vi "Beam Extraction.vi"() -> ()   [LabVIEW 2018]
uses:
  InstrumentStatusLib/com.insstat.lvlib
panel:
  out "?":bool
  out "?":bool
  out "?":bool
  out "?":bool
  out "?":string
  out "?":string
  out "?":string
  out "?":string
  out "?":bool
  out "?":bool
  out "?":bool
  out "?":bool
  out "?":string
  out "?":string
  out "?":string
  out "?":string
  out "Gate C":string
  out "Gate A":string
  out "REF":string
  out "Trig":string
  out "Gate B":string
  out "OUT":string
  out "Gate":string
  out "EN":string
  out "CS":string
  out "Pulse":string
  out "?":string
  out "?":string
  out "?":string
  out "?":string
  out "?":string
  out "?":string
  out "?":string
  out "?":string
  out "?":string
  out "?":string
  out "String":string
  out "?":string
  out "?":string
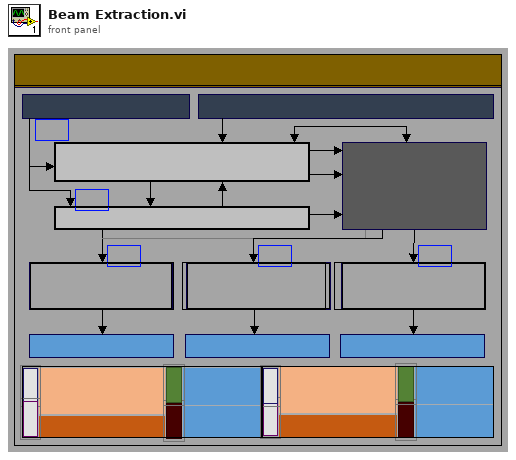
[diagram p1: front panel]
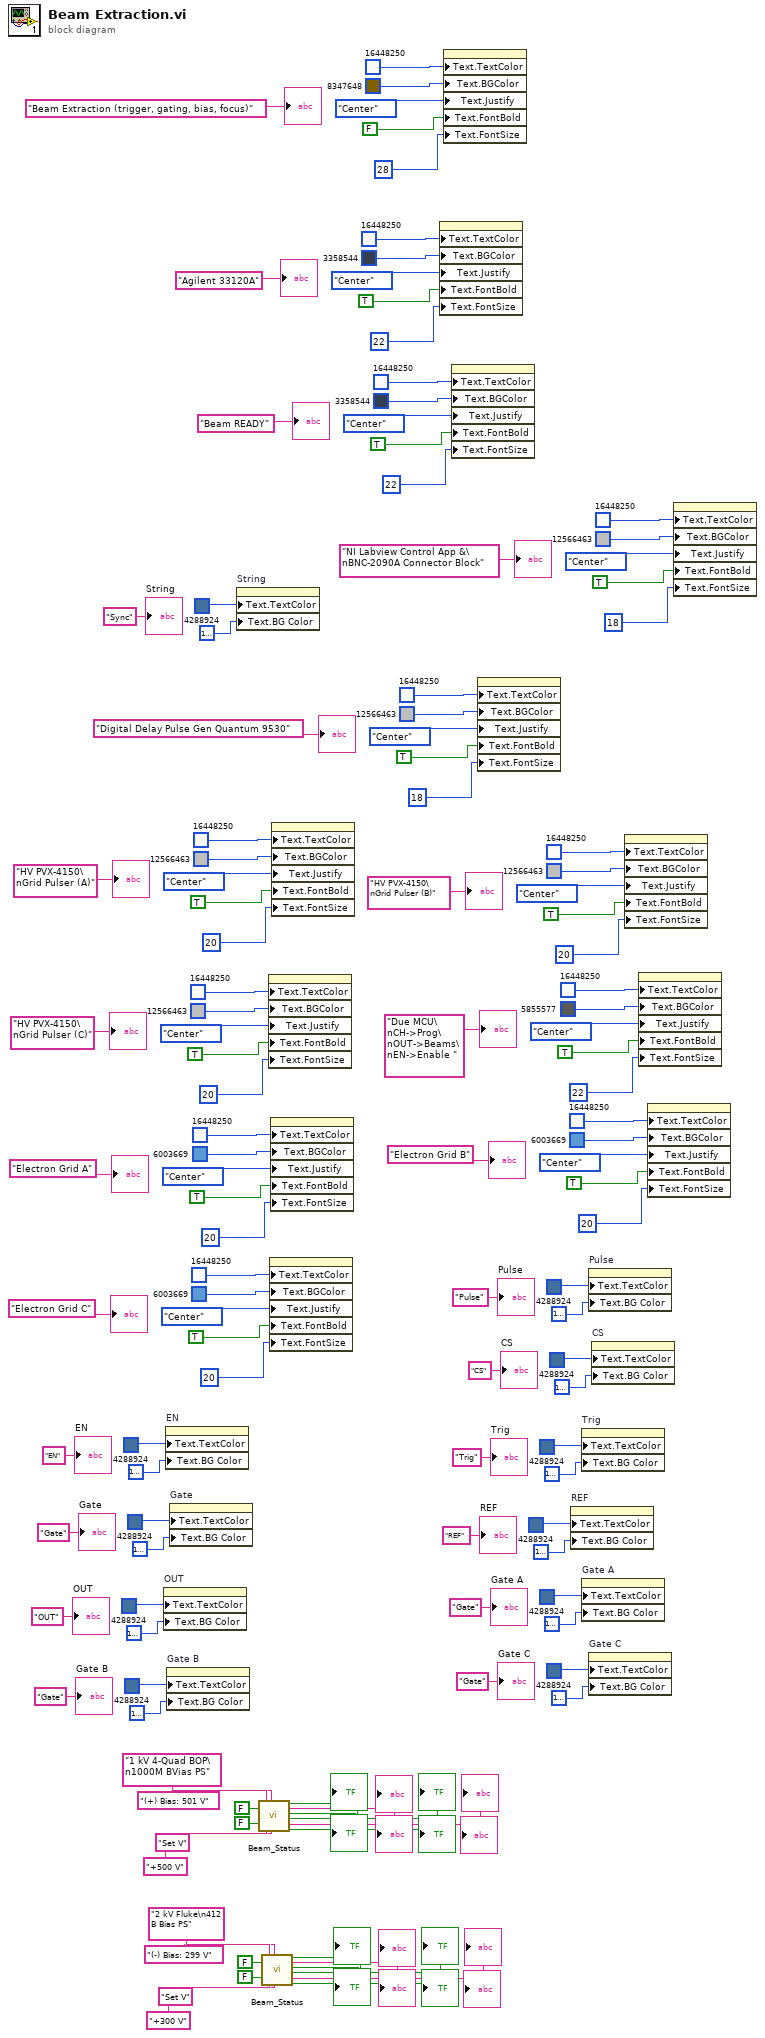
[diagram p0: block diagram]
diagram:
  n1 = property on="OUT" class="Str"("Text.TextColor"=u32 4288924, "Text.BG Color"=u32 16777216) -> ()  [unwired: 2 in, 2 out]
  n2 = property on="EN" class="Str"("Text.TextColor"=u32 4288924, "Text.BG Color"=u32 16777216) -> ()  [unwired: 2 in, 2 out]
  n3 = property on="Gate B" class="Str"("Text.TextColor"=u32 4288924, "Text.BG Color"=u32 16777216) -> ()  [unwired: 2 in, 2 out]
  n4 = property on="Gate" class="Str"("Text.TextColor"=u32 4288924, "Text.BG Color"=u32 16777216) -> ()  [unwired: 2 in, 2 out]
  n5 = property on="String" class="Str"("Text.TextColor"=u32 4288924, "Text.BG Color"=u32 16777216) -> ()  [unwired: 2 in, 2 out]
  n6 = call "Beam_Status.vi"("Power"=FALSE, "Activate"=FALSE, "String"="1 kV 4-Quad BOP\n1000M BVias PS", "String 3"="Set V", "String 2"="(+) Bias: 501 V", "String 4"="+500 V") -> (10:→"?":string, 11:→"?":string, 12:→"?":string, 13:→"?":string, 14:→"?":bool, 16:→"?":bool, 17:→"?":bool, 19:→"?":bool)  [unwired: 6 in]
  n7 = call "Beam_Status.vi"("Power"=FALSE, "Activate"=FALSE, "String"="2 kV Fluke\n412 B Bias PS", "String 3"="Set V", "String 2"="(-) Bias: 299 V", "String 4"="+300 V") -> (10:→"?":string, 11:→"?":string, 12:→"?":string, 13:→"?":string, 14:→"?":bool, 16:→"?":bool, 17:→"?":bool, 19:→"?":bool)  [unwired: 6 in]
  n8 = property class="Str"("Text.TextColor"=u32 16448250, "Text.BGColor"=u32 12566463, "Text.Justify"=enum16{"Left", "Center", "Right"}."Center" ("Text.Justification"), "Text.FontBold"=TRUE ("Text.Font:Bold"), "Text.FontSize"=u32 20 ("Text.Font:Size")) -> ()  [unwired: 2 in, 2 out]
  n9 = property class="Str"("Text.TextColor"=u32 16448250, "Text.BGColor"=u32 6003669, "Text.Justify"=enum16{"Left", "Center", "Right"}."Center" ("Text.Justification"), "Text.FontBold"=TRUE ("Text.Font:Bold"), "Text.FontSize"=u32 20 ("Text.Font:Size")) -> ()  [unwired: 2 in, 2 out]
  n10 = property class="Str"("Text.TextColor"=u32 16448250, "Text.BGColor"=u32 6003669, "Text.Justify"=enum16{"Left", "Center", "Right"}."Center" ("Text.Justification"), "Text.FontBold"=TRUE ("Text.Font:Bold"), "Text.FontSize"=u32 20 ("Text.Font:Size")) -> ()  [unwired: 2 in, 2 out]
  n11 = property class="Str"("Text.TextColor"=u32 16448250, "Text.BGColor"=u32 12566463, "Text.Justify"=enum16{"Left", "Center", "Right"}."Center" ("Text.Justification"), "Text.FontBold"=TRUE ("Text.Font:Bold"), "Text.FontSize"=u32 20 ("Text.Font:Size")) -> ()  [unwired: 2 in, 2 out]
  n12 = property class="Str"("Text.TextColor"=u32 16448250, "Text.BGColor"=u32 3358544, "Text.Justify"=enum16{"Left", "Center", "Right"}."Center" ("Text.Justification"), "Text.FontBold"=TRUE ("Text.Font:Bold"), "Text.FontSize"=u32 22 ("Text.Font:Size")) -> ()  [unwired: 2 in, 2 out]
  n13 = property class="Str"("Text.TextColor"=u32 16448250, "Text.BGColor"=u32 8347648, "Text.Justify"=enum16{"Left", "Center", "Right"}."Center" ("Text.Justification"), "Text.FontBold"=FALSE ("Text.Font:Bold"), "Text.FontSize"=u32 28 ("Text.Font:Size")) -> ()  [unwired: 2 in, 2 out]
  n14 = property class="Str"("Text.TextColor"=u32 16448250, "Text.BGColor"=u32 3358544, "Text.Justify"=enum16{"Left", "Center", "Right"}."Center" ("Text.Justification"), "Text.FontBold"=TRUE ("Text.Font:Bold"), "Text.FontSize"=u32 22 ("Text.Font:Size")) -> ()  [unwired: 2 in, 2 out]
  n15 = property class="Str"("Text.TextColor"=u32 16448250, "Text.BGColor"=u32 12566463, "Text.Justify"=enum16{"Left", "Center", "Right"}."Center" ("Text.Justification"), "Text.FontBold"=TRUE ("Text.Font:Bold"), "Text.FontSize"=u32 18 ("Text.Font:Size")) -> ()  [unwired: 2 in, 2 out]
  n16 = property on="REF" class="Str"("Text.TextColor"=u32 4288924, "Text.BG Color"=u32 16777216) -> ()  [unwired: 2 in, 2 out]
  n17 = property on="Trig" class="Str"("Text.TextColor"=u32 4288924, "Text.BG Color"=u32 16777216) -> ()  [unwired: 2 in, 2 out]
  n18 = property on="Gate A" class="Str"("Text.TextColor"=u32 4288924, "Text.BG Color"=u32 16777216) -> ()  [unwired: 2 in, 2 out]
  n19 = property on="Pulse" class="Str"("Text.TextColor"=u32 4288924, "Text.BG Color"=u32 16777216) -> ()  [unwired: 2 in, 2 out]
  n20 = property on="Gate C" class="Str"("Text.TextColor"=u32 4288924, "Text.BG Color"=u32 16777216) -> ()  [unwired: 2 in, 2 out]
  n21 = property on="CS" class="Str"("Text.TextColor"=u32 4288924, "Text.BG Color"=u32 16777216) -> ()  [unwired: 2 in, 2 out]
  n22 = property class="Str"("Text.TextColor"=u32 16448250, "Text.BGColor"=u32 12566463, "Text.Justify"=enum16{"Left", "Center", "Right"}."Center" ("Text.Justification"), "Text.FontBold"=TRUE ("Text.Font:Bold"), "Text.FontSize"=u32 20 ("Text.Font:Size")) -> ()  [unwired: 2 in, 2 out]
  n23 = property class="Str"("Text.TextColor"=u32 16448250, "Text.BGColor"=u32 5855577, "Text.Justify"=enum16{"Left", "Center", "Right"}."Center" ("Text.Justification"), "Text.FontBold"=TRUE ("Text.Font:Bold"), "Text.FontSize"=u32 22 ("Text.Font:Size")) -> ()  [unwired: 2 in, 2 out]
  n24 = property class="Str"("Text.TextColor"=u32 16448250, "Text.BGColor"=u32 6003669, "Text.Justify"=enum16{"Left", "Center", "Right"}."Center" ("Text.Justification"), "Text.FontBold"=TRUE ("Text.Font:Bold"), "Text.FontSize"=u32 20 ("Text.Font:Size")) -> ()  [unwired: 2 in, 2 out]
  n25 = property class="Str"("Text.TextColor"=u32 16448250, "Text.BGColor"=u32 12566463, "Text.Justify"=enum16{"Left", "Center", "Right"}."Center" ("Text.Justification"), "Text.FontBold"=TRUE ("Text.Font:Bold"), "Text.FontSize"=u32 18 ("Text.Font:Size")) -> ()  [unwired: 2 in, 2 out]
  "?" <- "Beam Extraction (trigger, gating, bias, focus)" ("String")
  "?" <- "Agilent 33120A" ("String")
  "?" <- "Beam READY" ("String")
  "String" <- "Sync" ("String")
  "?" <- "NI Labview Control App &\nBNC-2090A Connector Block"
  "?" <- "Digital Delay Pulse Gen Quantum 9530"
  "?" <- "HV PVX-4150\nGrid Pulser (A)"
  "?" <- "HV PVX-4150\nGrid Pulser (B)"
  "?" <- "HV PVX-4150\nGrid Pulser (C)"
  "?" <- "Due MCU\nCH->Prog\nOUT->Beams\nEN->Enable "
  "?" <- "Electron Grid A"
  "?" <- "Electron Grid B"
  "?" <- "Electron Grid C"
  "Pulse" <- "Pulse" ("String")
  "CS" <- "CS" ("String")
  "EN" <- "EN" ("String")
  "Gate" <- "Gate" ("String")
  "OUT" <- "OUT" ("String")
  "Gate B" <- "Gate" ("String")
  "Trig" <- "Trig" ("String")
  "REF" <- "REF" ("String")
  "Gate A" <- "Gate" ("String")
  "Gate C" <- "Gate" ("String")
